vi "Startup.vi"(7 "IP Address (localhost)":string, 8 "error in (no error)":errorcluster, 9 "max connections (0: no limit)":u32, 10 "TCP port (50007)":u16=50007) -> (0 "error out":errorcluster, 3 "JKI_Python_Server out":refnum<class "Server.lvclass">)   [LabVIEW 2013, in "JKI_Python_Bridge_for_LV.lvlib" / "Server.lvclass"]
uses:
  Server.lvclass
  Type Definitions/Class Private Data - Cluster.ctl
  <vilib>/addons/_JKI.lib/_jki_lib_tcp_server.llb/TCP Server Object RefNum__jki_lib_tcp_server.ctl
  <vilib>/addons/_JKI.lib/_jki_lib_tcp_server.llb/TCP Server Object RefNum - Enum__jki_lib_tcp_server.ctl
  Type Definitions/Python Node.ctl
  Call/Call.lvclass
  PyObject/PyObject.lvclass
  Type Definitions/Public Events - Cluster.ctl
  Server.lvclass/Server.ctl
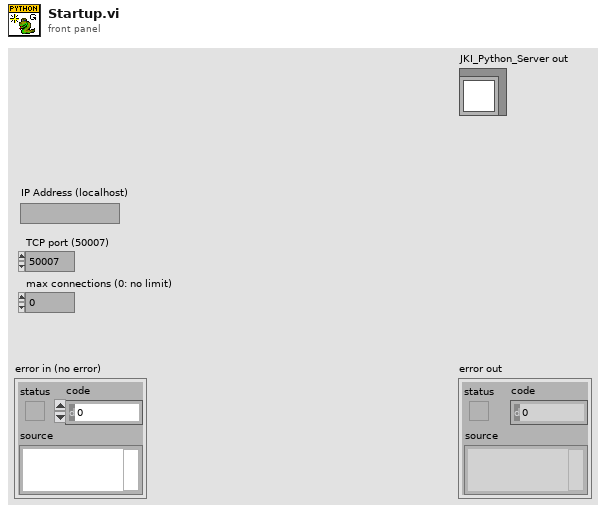
[diagram p1: front panel]
types:
  T1 = enum32{"invalid app kind", "Development System", "Run Time System", "Student Edition", "Embedded LabVIEW", "Evaluation", "Custom"}
  T2 = typedef "JKI_Python_Bridge_for_LV.lvlib/Server.lvclass/Class Private Data - Cluster.ctl" = cluster{"TCP Server RefNum":T3, "TCP port (50007)":u16, "max connections (0: no limit)":u32, "net address (0: Listen on All Adaptors)":u32, "Nodes":T4[], "Public Events":T5}
  T3 = typedef "TCP Server Object RefNum__jki_lib_tcp_server.ctl" = refnum<k1>
  T4 = typedef "JKI_Python_Bridge_for_LV.lvlib/Server.lvclass/Python Node.ctl" = cluster{"Name":string, "Python Method Call":refnum<user-event>, "Call Handle":refnum<class "PyObject.lvclass">}
  T5 = typedef "JKI_Python_Bridge_for_LV.lvlib/Server.lvclass/Public Events - Cluster.ctl" = cluster{"Stop Nodes":refnum<user-event>}
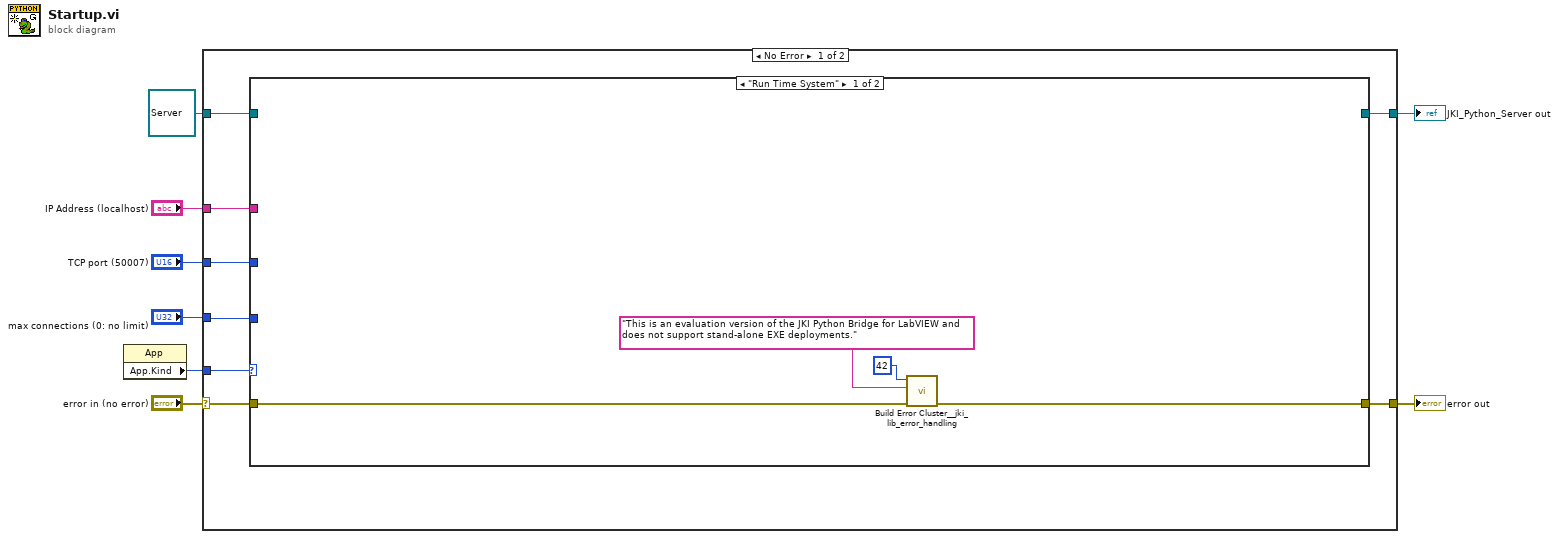
[diagram p0: block diagram]
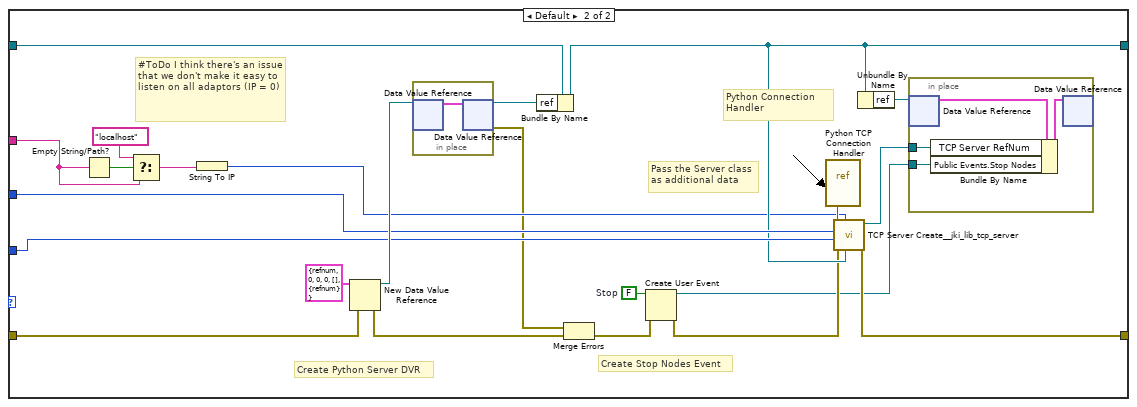
[diagram p2: hidden frame]
diagram:
  n1 = property class="App"() -> ("App.Kind"=w1:T1)  [unwired: 2 in, 2 out]
  n2 = case shown="No Error" "error in (no error)" {
    selector: "error in (no error)" -> [w16 w50]
    tunnel: [w12 w50] -> w7
    tunnel: [w11 w49] -> w5
    tunnel: refnum<class "Server.lvclass"> refnum ("JKI_Python_Server in") -> [w15 w49]
    tunnel: "TCP port (50007)" -> [w13 _]
    tunnel: "max connections (0: no limit)" -> [w14 _]
    tunnel: "IP Address (localhost)" -> [w10 _]
    tunnel: w1 -> [w9 _]
    frame No Error {
      n3 = case shown="\"Run Time System\"" w9 {
        tunnel: w16 -> [w20 w42]
        tunnel: w15 -> [_ w40]
        tunnel: w14 -> [_ w37]
        tunnel: w13 -> [_ w36]
        tunnel: [w19 w35] -> w12
        tunnel: [_ w33] -> w11
        tunnel: w10 -> [_ w29]
        frame "Run Time System" {
          n4 = call <vilib>:"Build Error Cluster__jki_lib_error_handling.vi"("error in"=w20, "String to Prepend to source (\"\")"="This is an evaluation version of the JKI Python Bridge for LabVIEW and does not support stand-alone EXE deployments." ("String to Prepend to source (\"\")"), "code"=42) -> ("error out"=w19:errorcluster)  [unwired: 8 in]
        }
        frame Default {
          w23 = FALSE  # Stop
          # "#ToDo I think there's an issue that we don't make it easy to listen on all adaptors (IP = 0)"
          # "Create Stop Nodes Event"
          # "Create Python Server DVR"
          # "Pass the Server class\nas additional data"
          # "Python Connection \nHandler"
          n5 = Empty String/Path?(string/path=w29) -> (empty?=w21:bool)
          n6 = Select(t="localhost" ("f"), s=w21, f=w29) -> (s? t:f=w28:string)
          n7 = String To IP(1:w28) -> (0:w31:u32)
          n8 = New Data Value Reference(data value=T2 {"TCP Server RefNum"=refnum, "TCP port (50007)"=0, "max connections (0: no limit)"=0, "net address (0: Listen on All Adaptors)"=0, "Nodes"=[], "Public Events"={"Stop Nodes"=refnum}} ("Private Data"), error in=w42) -> (data value reference=w41:refnum<data-value>, error out=w26:errorcluster)
          n9 = in-place {
            n10 = in-place-dvr #1(w41) -> (w48:T2)  [unwired: 1 out]
            n11 = in-place-dvr #1(w48) -> (w39:refnum<data-value>, w27:errorcluster)
          }
          n12 = Bundle By Name(cluster=w40, "ref"=w39) -> (w33:refnum<class "Server.lvclass">)
          n13 = Merge Errors(w27, w26) -> (w25:errorcluster)
          n14 = Create User Event(user event datatype=w23, error in=w25) -> (user event=w22:refnum<user-event>, error out=w24:errorcluster)
          n15 = vi-ref "Python TCP Connection Handler.vi"() -> ("vi reference"=w38:refnum<vi>)
          n16 = call <vilib>:"TCP Server Create__jki_lib_tcp_server.vi"("Additional Data"=w33, "net address (0: Listen on All Adaptors)"=w31, "error in (no error)"=w24, "max connections (0: no limit)"=w37, "port"=w36, "Connection Handler Call-Back VI RefNum"=w38) -> ("error out"=w35:errorcluster, "TCP Server RefNum"=w34:T3)  [unwired: 4 out]
          n17 = Unbundle By Name(w33) -> ("ref"=w32:refnum<data-value>)
          n18 = in-place {
            in-place-border: w34 -> [w47]
            in-place-border: w22 -> [w44]
            n19 = in-place-dvr #2(w32) -> (w46:T2)  [unwired: 1 out]
            n20 = Bundle By Name(cluster=w46, "TCP Server RefNum"=w47, "Public Events.Stop Nodes"=w44) -> (w45:T2)
            n21 = in-place-dvr #2(w45) -> ()  [unwired: 2 out]
          }
        }
      }
    }
    frame Error {
    }
  }
  "error out" <- w7
  "JKI_Python_Server out" <- w5
